vi "Read RTD_Parameter.vi"(8 "error in (no error)":errorcluster, 11 "PRM in":refnum<class "PRM.lvclass">) -> (0 "error out":errorcluster, 2 "RTD Parameter":T1={"A"=0.003809999907389283, "B"=-6.020000000717118e-07, "C"=-5.999999976025183e-12, "R0"=1000.0}, 3 "PRM out":refnum<class "PRM.lvclass">)   [LabVIEW 2019, in "PRM.lvlib" / "PRM.lvclass"]
uses:
  Library/PRM.lvclass
  Custom Controls/RTD Parameters.ctl
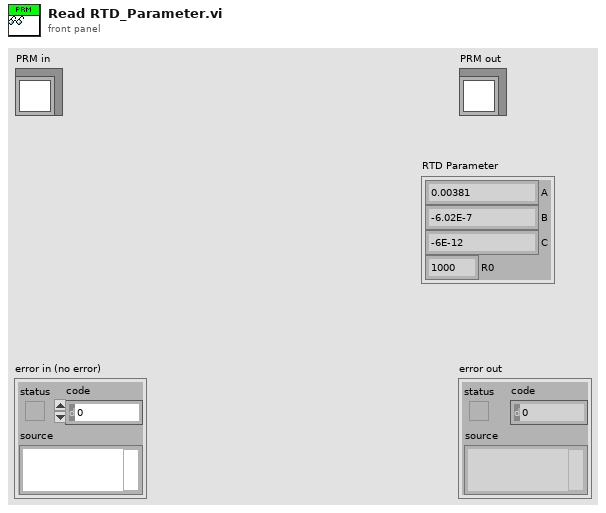
[diagram p1: front panel]
types:
  T1 = typedef "PRM.lvlib/PRM.lvclass/RTD Parameters.ctl" = cluster{"A":dbl, "B":dbl, "C":dbl, "R0":dbl}
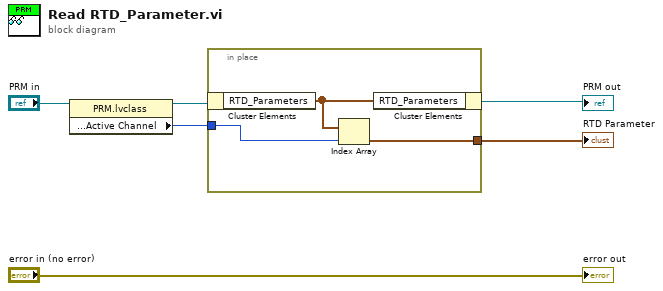
[diagram p0: block diagram]
diagram:
  n1 = property class="PRM.lvclass"(reference="PRM in") -> (reference out=w5:refnum<class "PRM.lvclass">, "Accessors:Settings:Active Channel"=w3:u32)  [unwired: 1 in, 1 out]
  n2 = in-place {
    in-place-border: w3 -> [w8]
    in-place-border: [w7] -> w2
    n3 = in-place-cluster #1(w5) -> ("RTD_Parameters"=w9:T1[])
    n4 = Index Array(array=w9, index=w8) -> (element=w7:T1)
    n5 = in-place-cluster #1("RTD_Parameters"=w9) -> (→"PRM out":refnum<class "PRM.lvclass">)
  }
  "RTD Parameter" <- w2
  "error out" <- "error in (no error)"
